vi "Checkin.vi"(8 "error in (no error)":errorcluster, 9 "Timeout(-1)":dbl[unit], 10 "Object":refnum<class "CS++Base.lvclass">, 11 "Object Reference":refnum<class "CS++Reference.lvclass">) -> (0 "error out":errorcluster, 1 "timed out?":bool, 3 "Object Reference out":refnum<class "CS++Reference.lvclass">)   [LabVIEW 2013, in "CS++BaseClasses.lvlib" / "CS++Reference.lvclass"]
doc: "Checkin object into Reference."
uses:
  CS++Reference.lvclass
  Base/CS++Base.lvclass
  CS++Reference.lvclass/CS++Reference.ctl
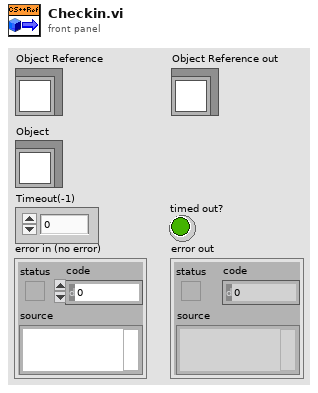
[diagram p1: front panel]
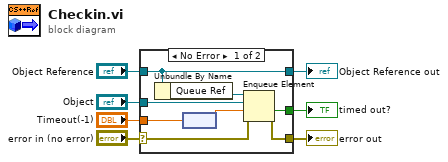
[diagram p0: block diagram]
diagram:
  n1 = case shown="No Error" "error in (no error)" {
    selector: "error in (no error)" -> [w10 w17]
    tunnel: [w9 w17] -> w6
    tunnel: [w15 w16] -> w4
    tunnel: "Object Reference" -> [w15 w16]
    tunnel: "Object" -> [w13 _]
    tunnel: "Timeout(-1)" -> [w11 _]
    tunnel: [w8 _] -> w1
    frame No Error {
      n2 = Unbundle By Name(w15) -> ("Queue Ref"=w14:refnum<queue>)
      n3 = node(w11) -> (w12:dbl)
      n4 = Enqueue Element(queue=w14, element=w13, timeout in ms (-1)=w12, error in (no error)=w10) -> (timed out?=w8:bool, error out=w9:errorcluster)  [unwired: 1 out]
    }
    frame Error {
    }
  }
  "error out" <- w6
  "Object Reference out" <- w4
  "timed out?" <- w1
